vi "user2.vi"() -> ()   [LabVIEW 2017]
uses:
  people.ctl
panel:
  in  "To":T1
  in  "From":T1
  out "error out":errorcluster
  in  "error in":errorcluster
  out "Messages":string
  in  "EXIT":bool
  in  "SEND":bool
  in  "Message":string
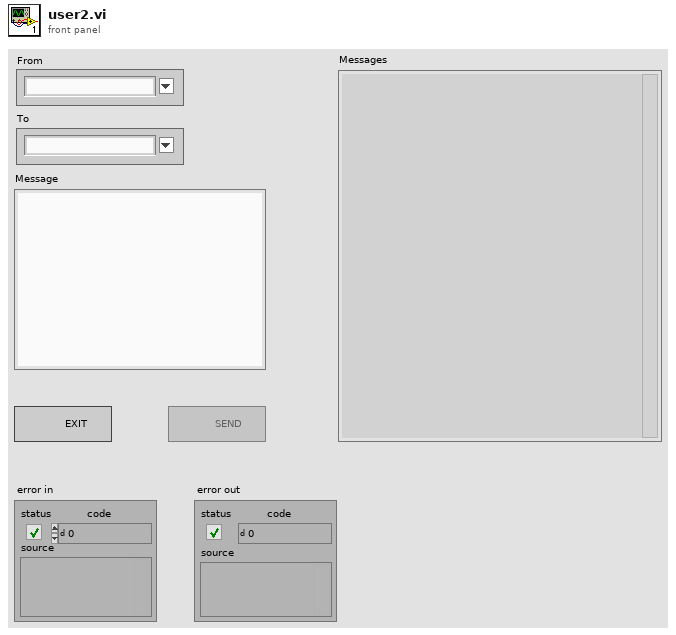
[diagram p1: front panel]
types:
  T1 = typedef "people.ctl" = string
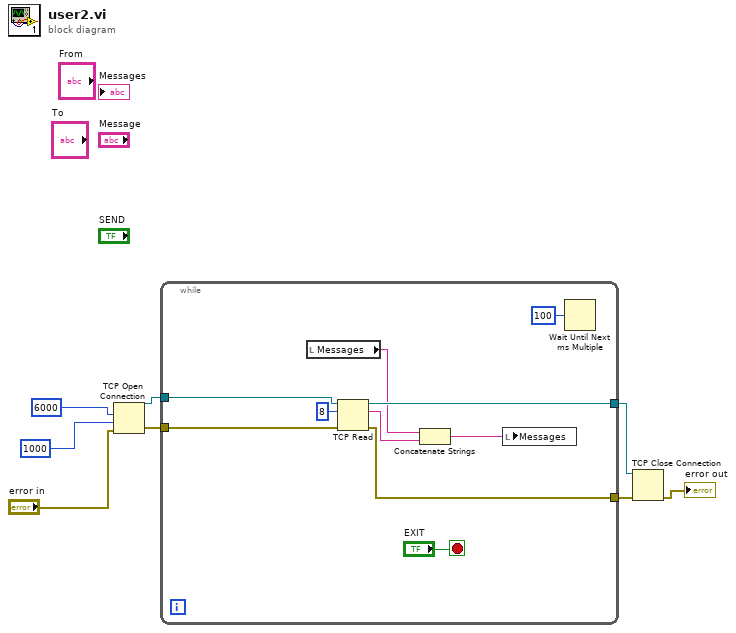
[diagram p0: block diagram]
diagram:
  n1 = TCP Open Connection(remote port or service name=u16 6000, timeout ms (60000)=1000, error in (no error)="error in") -> (connection ID=w4:refnum<k5>, error out=w3:errorcluster)  [unwired: 2 in]
  n2 = while {
    tunnel: [w17] -> w7
    tunnel: [w16] -> w6
    tunnel: w4 -> [w15]
    tunnel: w3 -> [w11]
    stop <- "EXIT" stop-if-true
    n3 = local read "Messages"() -> (w14:string)
    n4 = TCP Read(connection ID=w15, bytes to read=8, error in (no error)=w11) -> (connection ID out=w17:refnum<k5>, data out=w12:string, error out=w16:errorcluster)  [unwired: 2 in]
    n5 = Concatenate Strings "Concatenate Strings"(w14, w12) -> (w13:string)
    n6 = local write "Messages"(w13) -> ()
    n7 = Wait Until Next ms Multiple(millisecond multiple=u32 100) -> ()  [unwired: 1 out]
  }
  n8 = TCP Close Connection(connection ID=w7, error in (no error)=w6) -> (error out=→"error out":errorcluster)  [unwired: 1 in, 1 out]
